vi "p2.vi"() -> ()   [LabVIEW 2021, in "d8.lvlib"]
uses:
  d8.lvlib
  AOC/AOC.lvlib
panel:
  in  "Example":string="30373\n25512\n65332\n33549\n35390"
  in  "Example":bool
  out "Answer":i64=590824
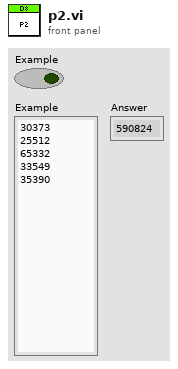
[diagram p1: front panel]
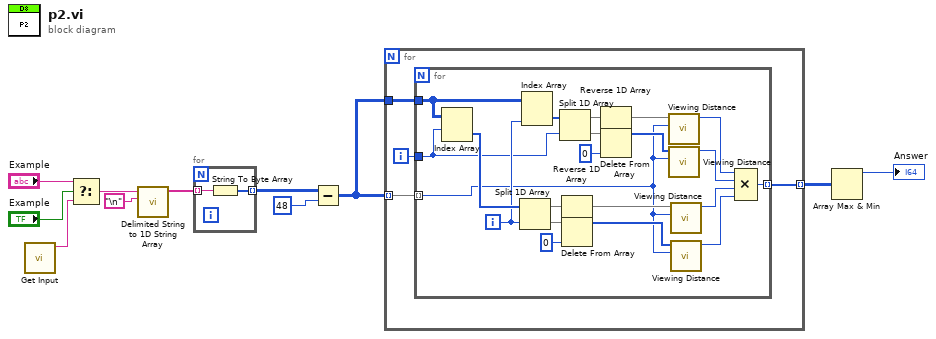
[diagram p0: block diagram]
diagram:
  n1 = call "Get Input.vi"() -> ("Input"=w11:string)  [unwired: 11 in]
  n2 = Select(t="Example", s="Example", f=w11) -> (s? t:f=w10:string)
  n3 = call <vilib>:"Delimited String to 1D String Array.vi"("delimiter"="\n", "delimited string"=w10) -> ("string array"=w4:string[])  [unwired: 9 in]
  n4 = for {
    tunnel: w4 -> [w13] mode=indexing
    tunnel: [w12] -> w6 mode=indexing
    n5 = String To Byte Array(string=w13) -> (unsigned byte array=w12:u8[])
  }
  n6 = Subtract(x=w6, y=u8 48) -> (x-y=w3:u8[][])
  n7 = for {
    tunnel: w3 -> [w17] mode=indexing
    tunnel: w3 -> [w16]
    tunnel: [w14] -> w2 mode=indexing
    i -> [w15]
    n8 = for {
      tunnel: w17 -> [w23] mode=indexing
      tunnel: w16 -> [w38]
      tunnel: w15 -> [w32]
      tunnel: [w18] -> w14 mode=indexing
      i -> [w36]
      n9 = Index Array(array=w38, index (row)=w32) -> (element=w37:u8[])  [unwired: 1 in]
      n10 = Split 1D Array(array=w37, index=w36) -> (first subarray=w29:u8[], second subarray=w34:u8[])
      n11 = Index Array(array=w38, index (col)=w36) -> (element=w33:u8[])  [unwired: 1 in]
      n12 = Split 1D Array(array=w33, index=w32) -> (first subarray=w28:u8[], second subarray=w30:u8[])
      n13 = Reverse 1D Array(array=w29) -> (reversed array=w27:u8[])
      n14 = Delete From Array(array=w34, index=0) -> (array with subset deleted=w26:u8[])  [unwired: 1 in, 1 out]
      n15 = Reverse 1D Array(array=w28) -> (reversed array=w24:u8[])
      n16 = Delete From Array(array=w30, index=0) -> (array with subset deleted=w25:u8[])  [unwired: 1 in, 1 out]
      n17 = call "Viewing Distance.vi"("Tree"=w23, "Trees"=w24) -> ("NTrees"=w22:i64)  [unwired: 9 in]
      n18 = call "Viewing Distance.vi"("Tree"=w23, "Trees"=w25) -> ("NTrees"=w21:i64)  [unwired: 9 in]
      n19 = call "Viewing Distance.vi"("Tree"=w23, "Trees"=w27) -> ("NTrees"=w20:i64)  [unwired: 9 in]
      n20 = call "Viewing Distance.vi"("Tree"=w23, "Trees"=w26) -> ("NTrees"=w19:i64)  [unwired: 9 in]
      n21 = Compound Arithmetic op=MULTIPLY(w22, w21, w20, w19) -> (w18:i64)
    }
  }
  n22 = Array Max & Min(array=w2) -> (max value=→"Answer":i64)  [unwired: 3 out]
